vi "Enqueue Single Element.vi"(6 "Priority":T2, 8 "error in (no error)":errorcluster, 10 "Message":T1, 11 "QDMH in":refnum<class "QDMH.lvclass">) -> (0 "error out":errorcluster, 3 "QDMH out":refnum<class "QDMH.lvclass">)   [LabVIEW 2023, in "QDMH.lvlib" / "QDMH.lvclass"]
doc: "Enqueue Fully Formed message with data\nPriority determines if the item is enqueued at the end of the stack or the front:\n\nLow: Add to End\nHigh: Add to front"
uses:
  Library/QDMH.lvclass
  Custom Controls/Enqueue Priority.ctl
  Custom Controls/Message.ctl
  Library/QDMH.lvclass/QDMH.ctl
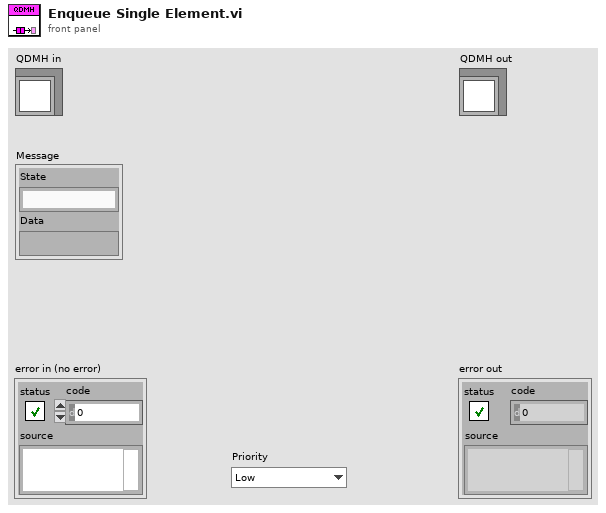
[diagram p1: front panel]
types:
  T1 = typedef "QDMH.lvlib/QDMH.lvclass/Message.ctl" = cluster{"State":string, "Data":variant}
  T2 = typedef "QDMH.lvlib/QDMH.lvclass/Enqueue Priority.ctl" = enum16{"Low", "High"}
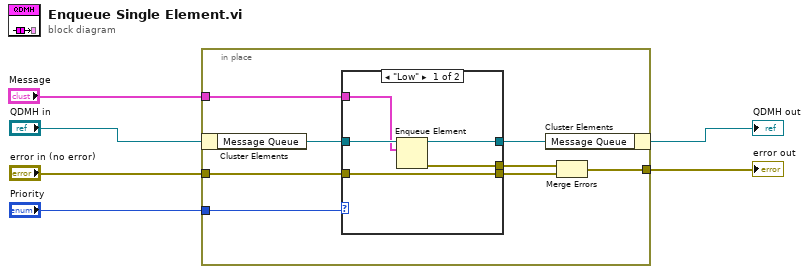
[diagram p0: block diagram]
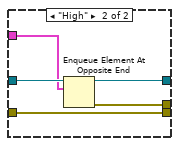
[diagram p2: hidden frame]
diagram:
  n1 = in-place {
    in-place-border: "Priority" -> [w14]
    in-place-border: [w8] -> w3
    in-place-border: "error in (no error)" -> [w10]
    in-place-border: "Message" -> [w9]
    n2 = in-place-cluster #1("QDMH in") -> ("Message Queue"=w13:refnum<queue>)
    n3 = case shown="\"Low\"" w14 {
      tunnel: w13 -> [w19 w24]
      tunnel: [w18 w23] -> w12
      tunnel: [w17 w22] -> w11
      tunnel: w10 -> [w15 w20]
      tunnel: w9 -> [w16 w21]
      tunnel: [w15 w20] -> w7
      frame "Low" {
        n4 = Enqueue Element(queue=w19, element=w16) -> (queue out=w18:refnum<queue>, error out=w17:errorcluster)  [unwired: 2 in, 1 out]
      }
      frame "High" {
        n5 = Enqueue Element At Opposite End(queue=w24, element=w21) -> (queue out=w23:refnum<queue>, error out=w22:errorcluster)  [unwired: 2 in, 1 out]
      }
    }
    n6 = in-place-cluster #1("Message Queue"=w12) -> (→"QDMH out":refnum<class "QDMH.lvclass">)
    n7 = Merge Errors(w11, w7) -> (w8:errorcluster)
  }
  "error out" <- w3
